vi "disconnect.vi"(8 "error in (no error)":errorcluster, 11 "RabbitMQ Session In":T1) -> (0 "error out":errorcluster)   [LabVIEW 2019, in "rabbitmq.lvlib"]
uses:
  rabbitmq.lvlib
  session.ctl
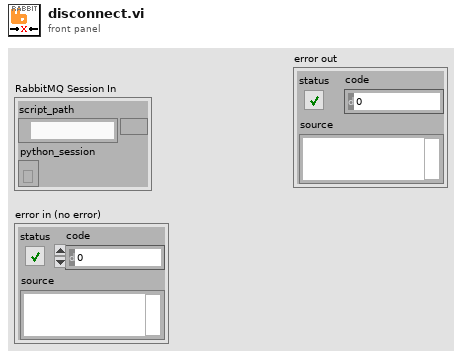
[diagram p1: front panel]
types:
  T1 = typedef "rabbitmq.lvlib/session.ctl" = cluster{"script_path":path, "python_session":refnum<k35>}
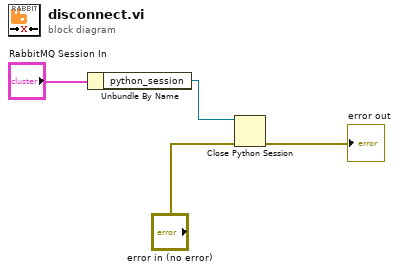
[diagram p0: block diagram]
diagram:
  n1 = Unbundle By Name("RabbitMQ Session In") -> ("python_session"=w3:refnum<k35>)
  n2 = Close Python Session(session in=w3, error in="error in (no error)") -> (11:→"error out":errorcluster)
